vi "Post-Build Action - Rename AppName Section.vi"(5 "Files Generated by Build":path[](array[path]), 6 "Top Level/Always Included VIs":path[](array[path]), 7 "Destination Path":path, 8 "error in (no error)":errorcluster, 9 "Target Name":string, 10 "Build Specification Name":string, 11 "Project Path":path) -> (0 "error out":errorcluster)   [LabVIEW 2015, in "Build Tools.lvlib"]
doc: "The purpose of this build action is to update the [AppName] section name in the main ini file so that it contains the name of the application."
uses:
  Build Tools.lvlib
  <userlib>/_OpenG.lib/file/file.llb/Convert File Extension (String)__ogtk.vi
panel:
  out "New INI contents":string
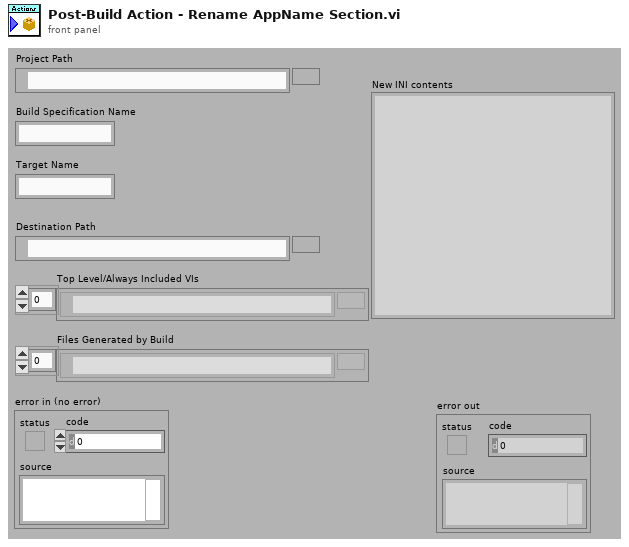
[diagram p1: front panel]
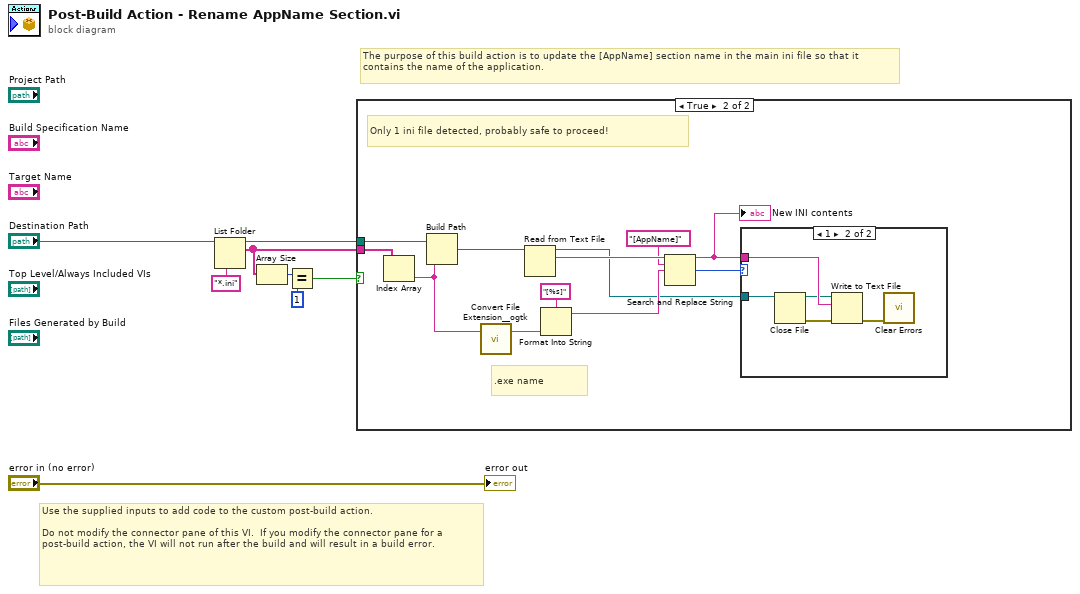
[diagram p0: block diagram]
diagram:
  # "The purpose of this build action is to update the [AppName] section name in the main ini file so that it contains the name of the application."
  # "Use the supplied inputs to add code to the custom post-build action.\n\nDo not modify the connector pane of this VI.  If you modify the connector pane for a post-build action, the VI will not run after the build and will result in a build error."
  n1 = List Folder(path="Destination Path", pattern="*.ini") -> (path out=w2:path, filenames=w1:string[])  [unwired: 2 in, 2 out]
  n2 = Array Size(array=w1) -> (size(s)=w5:i32)
  n3 = Equal?(x=w5, y=1) -> (x = y?=w3:bool)
  n4 = case shown="True" w3 {
    tunnel: w2 -> [_ w19]
    tunnel: w1 -> [_ w20]
    frame False {
      # "More than 1 ini file detected, probably not safe to proceed!"
    }
    frame True {
      # ".exe name"
      # "Only 1 ini file detected, probably safe to proceed!"
      n5 = Index Array(array=w20) -> (element=w9:string)  [unwired: 1 in]
      n6 = Build Path(base path=w19, name or relative path=w9) -> (appended path=w14:path)
      n7 = call-poly <userlib>:"Convert File Extension__ogtk.vi"("file name"=w9) -> ("new filename"=w13:string)  [unwired: 1 in, 1 out]
      n8 = Read from Text File(file (use dialog)=w14) -> (refnum out=w12:refnum<file>, text=w18:string)  [unwired: 3 in, 2 out]
      n9 = Format Into String(format string="[%s]", w13) -> (resulting string=w15:string)  [unwired: 2 in, 1 out]
      n10 = Search and Replace String(input string=w18, search string="[AppName]", replace string=w15) -> (result string=w11:string, number of replacements=w10:i32)  [unwired: 5 in, 2 out]
      "New INI contents" <- w11
      n11 = case shown="1" w10 {
        tunnel: w12 -> [_ w23]
        tunnel: w11 -> [_ w22]
        frame Default {
        }
        frame 1 {
          n12 = Close File(refnum=w23) -> (path=w21:path, error out=w25:errorcluster)  [unwired: 1 in]
          n13 = Write to Text File(file (use dialog)=w21, text=w22, error in=w25) -> (error out=w24:errorcluster)  [unwired: 1 in, 2 out]
          n14 = call <vilib>:"Clear Errors.vi"("error in (no error)"=w24) -> ()  [unwired: 5 in, 2 out]
        }
      }
    }
  }
  "error out" <- "error in (no error)"
